vi "Manage Indentation of Preset components.vi"(8 "error in (no error)":errorcluster, 11 "Tree Refnum":refnum<vi>) -> (0 "error out":errorcluster)   [LabVIEW 2012]
doc: "SciScan 1.2 160622"
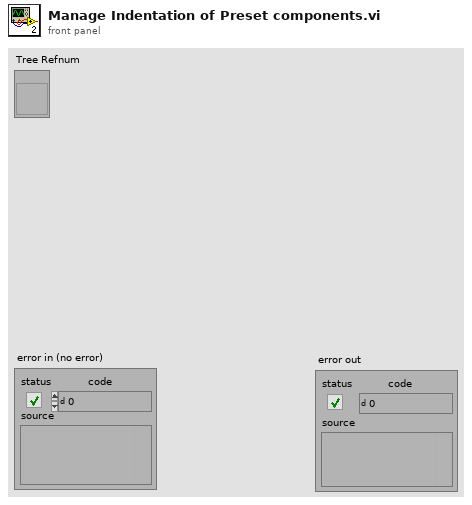
[diagram p1: front panel]
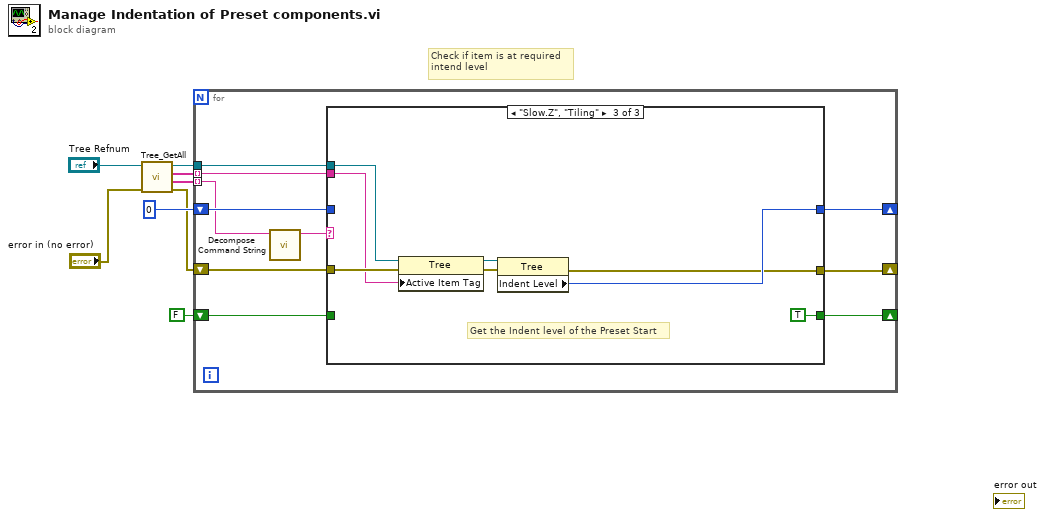
[diagram p0: block diagram]
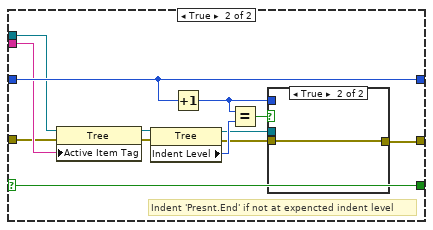
[diagram p3: hidden frame]
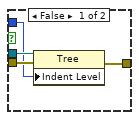
[diagram p4: hidden frame]
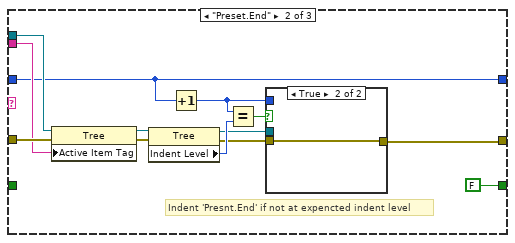
[diagram p5: hidden frame]
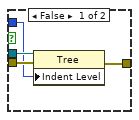
[diagram p6: hidden frame]
diagram:
  # "Check if item is at required\nintend level"
  n1 = call "Tree_GetAll.vi"("Error In"="error in (no error)", "Tree Refnum IN"="Tree Refnum") -> ("Error Out"=w2:errorcluster, "Text"=w1:string[], "Tags"=w7:string[], "Tree Refnum OUT"=w6:refnum<vi>)  [unwired: 6 in]
  n2 = for {
    tunnel: w6 -> [w17]
    tunnel: w7 -> [w11] mode=indexing
    shift-right: [w18] -> _
    shift-left: FALSE -> [w15]
    shift-right: [w16] -> _
    shift-left: 0 ("Indent Level") -> [w14]
    shift-right: [w12] -> _
    shift-left: w2 -> [w13]
    tunnel: w1 -> [w10] mode=indexing
    n3 = call "Decompose Command String.vi"("Command IN"=w10) -> ("Action"=w9:string)  [unwired: 7 in, 3 out]
    n4 = case shown="\"Slow.Z\", \"Tiling\"" w9 {
      tunnel: [w23 FALSE TRUE] -> w18
      tunnel: w17 -> [w21 w55 w71]
      tunnel: [w25 w54 w70] -> w16
      tunnel: w15 -> [w26 _ _]
      tunnel: w14 -> [w24 w54 _]
      tunnel: w13 -> [w19 w57 w69]
      tunnel: [w20 w48 w68] -> w12
      tunnel: w11 -> [w22 w56 w67]
      frame Default {
        n5 = case shown="False" w26 {
          selector: w26 -> [w28 w42]
          tunnel: [w29 w34] -> w25
          tunnel: w24 -> [w29 w34]
          tunnel: [w28 w42] -> w23
          tunnel: w22 -> [_ w32]
          tunnel: w21 -> [_ w33]
          tunnel: [w27 w30] -> w20
          tunnel: w19 -> [w27 w31]
          frame False {
          }
          frame True {
            # "Indent 'Presnt.End' if not at expencted indent level"
            n6 = property class="Tree"(reference=w33, error in=w31, "Active Item Tag"=w32) -> (reference out=w40:refnum<vi>, error out=w41:errorcluster)
            n7 = property class="Tree"(reference=w40, error in=w41) -> (reference out=w36:refnum<vi>, error out=w35:errorcluster, "Indent Level"=w39:i32)
            n8 = Increment(x=w34) -> (x+1=w37:i32)
            n9 = Equal?(x=w37, y=w39) -> (x = y?=w38:bool)
            n10 = case shown="True" w38 {
              tunnel: w37 -> [w44 _]
              tunnel: w36 -> [w46 _]
              tunnel: w35 -> [w45 w47]
              tunnel: [w43 w47] -> w30
              frame False {
                n11 = property class="Tree"(reference=w46, error in=w45, "Indent Level"=w44) -> (error out=w43:errorcluster)  [unwired: 1 out]
              }
              frame True {
              }
            }
          }
        }
      }
      frame "Preset.End" {
        # "Indent 'Presnt.End' if not at expencted indent level"
        n12 = property class="Tree"(reference=w55, error in=w57, "Active Item Tag"=w56) -> (reference out=w58:refnum<vi>, error out=w59:errorcluster)
        n13 = property class="Tree"(reference=w58, error in=w59) -> (reference out=w50:refnum<vi>, error out=w49:errorcluster, "Indent Level"=w53:i32)
        n14 = Increment(x=w54) -> (x+1=w51:i32)
        n15 = Equal?(x=w51, y=w53) -> (x = y?=w52:bool)
        n16 = case shown="True" w52 {
          tunnel: w51 -> [w62 _]
          tunnel: w50 -> [w64 _]
          tunnel: w49 -> [w63 w65]
          tunnel: [w61 w65] -> w48
          frame False {
            n17 = property class="Tree"(reference=w64, error in=w63, "Indent Level"=w62) -> (error out=w61:errorcluster)  [unwired: 1 out]
          }
          frame True {
          }
        }
      }
      frame "Slow.Z", "Tiling" {
        # "Get the Indent level of the Preset Start"
        n18 = property class="Tree"(reference=w71, error in=w69, "Active Item Tag"=w67) -> (reference out=w66:refnum<vi>, error out=w72:errorcluster)
        n19 = property class="Tree"(reference=w66, error in=w72) -> (error out=w68:errorcluster, "Indent Level"=w70:i32)  [unwired: 1 out]
      }
    }
  }
